vi "Read-Write Backspan Settings File.vi"(0 "configuration file path":path=path "C:/ProgramData/PVI Systems/Staple Inspection System/Measurement Settings.xml", 1 "Backplane Settings":T2={"Setup"={"Show Search Area"=FALSE, "Show Search Lines"=FALSE, "Show Edges Found"=FALSE, "Show Result"=FALSE}, "Outside Edge Options"={"Edge Polarity"=0, "Kernel Size"=13, "Width"=19, "Minimum Edge Strength"=100.0, "Interpolation Type"=enum."Zero Order", "Data Processing Method"=enum."Average"}, "Outside Line Options"={"Number of Lines"=1, "Type"=enum."First Edge Rake", "Min. Score"=0.0, "Max. Score"=1024.0, "Orientation"=0.0, "Angle Range"=40.0, "Angle Tolerance"=5.0, "Step Size"=20, "Min. SNR (db)"=0.0, "Min. Points (%)"=2.0, "Hough Iterations"=5}, "Settings Caliper"={"Contrast"=40, "Filter width"=4, "Steepness"=2, "Subsampling Ratio"=5, "Show Search Area"=FALSE, "Show Search Lines"=FALSE, "Show Edges Found"=FALSE, "Show Result"=FALSE}, "Look For (Bright Objects)"=1, "Method"=1, "Kernel Size"={"SizeX"=176, "SizeY"=176}, "Niblack Deviation Factor"=0.12, "Number of Erosion"=2, "Score Delineator"=150.0, "Auto Adjust Kernel Size"=TRUE, "Threshold Method"=0, "Use Quick method\nThreshold"=TRUE, "Scale Score"=TRUE, "Area Filter > 2"=10000.0, "Inside Edge Options"={"Edge Polarity"=1, "Kernel Size"=13, "Width"=19, "Minimum Edge Strength"=100.0, "Interpolation Type"=enum."Zero Order", "Data Processing Method"=enum."Average"}, "Inside Line Options"={"Number of Lines"=1, "Type"=enum."First Edge Rake", "Min. Score"=0.0, "Max. Score"=1024.0, "Orientation"=0.0, "Angle Range"=25.0, "Angle Tolerance"=1.0, "Step Size"=20, "Min. SNR (db)"=0.0, "Min. Points (%)"=1.0, "Hough Iterations"=5}, "Inner Width Reduce %"=5.0, "Inner Height Reduce %"=15.0, "Inner Setup"={"Show Search Area"=FALSE, "Show Search Lines"=FALSE, "Show Edges Found"=FALSE, "Show Result"=FALSE}, "Show CoM"=FALSE, "Keep All Results"=FALSE, "X Size"=0.0, "Y Size"=0.0, ">2 Holes % perimeter"=0.0, "Expected Backspan Width (Pixels)"=160, "Boundry Flex"=0.0, "Center Angle"=2.0} {"Inside Edge Options"."Edge Polarity" items=["All Edges", "Rising Edges", "Falling Edges"]; "Threshold Method" items=["clustering", "entropy", "metric", "moments", "inter-class variance"]; "Score Delineator" format="%#_15g"; "Niblack Deviation Factor" format="%#_15g"; "Method" items=["Niblack", "Background Correction"]; "Look For (Bright Objects)" items=["Bright Objects", "Dark Objects"]; "Outside Edge Options"."Edge Polarity" items=["All Edges", "Rising Edges", "Falling Edges"]}, 2 "Mode":T1=enum."Write", 3 "error in":errorcluster) -> (7 "Config File Path":path=path "C:/ProgramData/PVI Systems/Staple Inspection System/Config.ini", 8 "Backplane Settings Out":T2={"Setup"={"Show Search Area"=FALSE, "Show Search Lines"=FALSE, "Show Edges Found"=FALSE, "Show Result"=TRUE}, "Outside Edge Options"={"Edge Polarity"=0, "Kernel Size"=13, "Width"=19, "Minimum Edge Strength"=100.0, "Interpolation Type"=enum."Zero Order", "Data Processing Method"=enum."Average"}, "Outside Line Options"={"Number of Lines"=1, "Type"=enum."First Edge Rake", "Min. Score"=0.0, "Max. Score"=1024.0, "Orientation"=0.0, "Angle Range"=20.0, "Angle Tolerance"=1.0, "Step Size"=20, "Min. SNR (db)"=0.0, "Min. Points (%)"=2.0, "Hough Iterations"=5}, "Settings Caliper"={"Contrast"=40, "Filter width"=4, "Steepness"=2, "Subsampling Ratio"=5, "Show Search Area"=FALSE, "Show Search Lines"=FALSE, "Show Edges Found"=FALSE, "Show Result"=FALSE}, "Look For (Bright Objects)"=1, "Method"=1, "Kernel Size"={"SizeX"=176, "SizeY"=176}, "Niblack Deviation Factor"=0.2, "Number of Erosion"=2, "Score Delineator"=150.0, "Auto Adjust Kernel Size"=TRUE, "Threshold Method"=2, "Use Quick method\nThreshold"=TRUE, "Scale Score"=TRUE, "Area Filter > 2"=10000.0, "Inside Edge Options"={"Edge Polarity"=2, "Kernel Size"=13, "Width"=19, "Minimum Edge Strength"=100.0, "Interpolation Type"=enum."Zero Order", "Data Processing Method"=enum."Average"}, "Inside Line Options"={"Number of Lines"=1, "Type"=enum."First Edge Rake", "Min. Score"=0.0, "Max. Score"=1024.0, "Orientation"=0.0, "Angle Range"=25.0, "Angle Tolerance"=1.0, "Step Size"=20, "Min. SNR (db)"=0.0, "Min. Points (%)"=1.0, "Hough Iterations"=5}, "Inner Width Reduce %"=30.0, "Inner Height Reduce %"=15.0, "Inner Setup"={"Show Search Area"=FALSE, "Show Search Lines"=FALSE, "Show Edges Found"=FALSE, "Show Result"=TRUE}, "Show CoM"=FALSE, "Keep All Results"=FALSE, "X Size"=0.0, "Y Size"=0.0, ">2 Holes % perimeter"=0.0, "Expected Backspan Width (Pixels)"=140, "Boundry Flex"=0.0, "Center Angle"=0.0} {"Inside Edge Options"."Edge Polarity" items=["All Edges", "Rising Edges", "Falling Edges"]; "Threshold Method" items=["clustering", "entropy", "metric", "moments", "inter-class variance"]; "Score Delineator" format="%#_15g"; "Niblack Deviation Factor" format="%#_15g"; "Method" items=["Niblack", "Background Correction"]; "Look For (Bright Objects)" items=["Bright Objects", "Dark Objects"]; "Outside Edge Options"."Edge Polarity" items=["All Edges", "Rising Edges", "Falling Edges"]}, 10 "error out":errorcluster)   [LabVIEW 2013, in "Config Module.lvlib"]
uses:
  Config Module.lvlib
  Measurement Library/Controls/ASMS Backplane Settings Cluster.ctl
  Controls/Config File Operation Enum.ctl
  XML Config/XML Config.lvlib
  Measurement Library/Measurement Library.lvlib
panel:
  out "XML":string
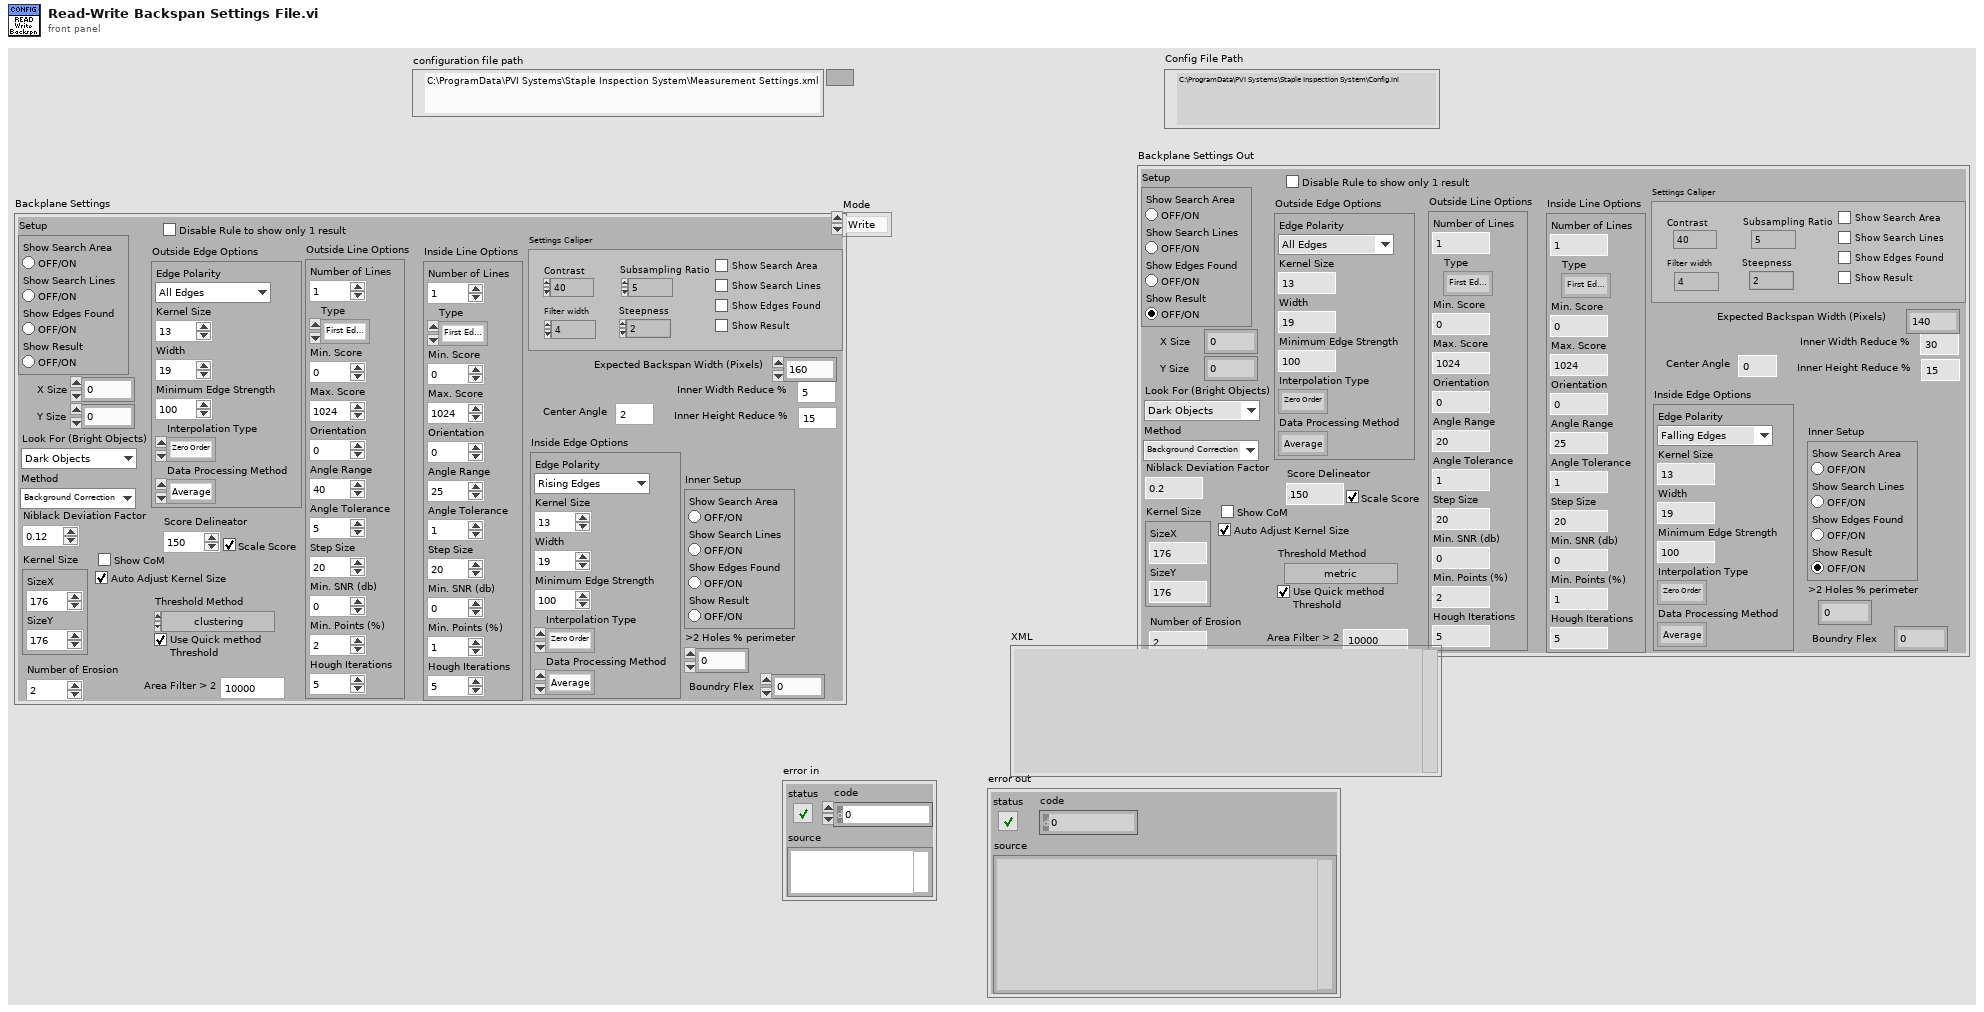
[diagram p1: front panel]
types:
  T1 = typedef "Config Module.lvlib/Config File Operation Enum.ctl" = enum16{"Read", "Write"}
  T2 = typedef "Measurement Library.lvlib/ASMS Backplane Settings Cluster.ctl" = cluster{"Setup":cluster{"Show Search Area":bool, "Show Search Lines":bool, "Show Edges Found":bool, "Show Result":bool}, "Outside Edge Options":cluster{"Edge Polarity":u32, "Kernel Size":u32, "Width":u32, "Minimum Edge Strength":sgl, "Interpolation Type":enum32{"Zero Order", "Bilinear", "Quadratic", "Cubic", "Bilinear Fixed"}, "Data Processing Method":enum32{"Average", "Median"}}, "Outside Line Options":cluster{"Number of Lines":i32, "Type":enum32{"First Edge Rake", "Best Edge Rake", "Hough Edge Rake", "First Edge Projection", "Best Edge Projection"}, "Min. Score":dbl, "Max. Score":dbl, "Orientation":dbl, "Angle Range":dbl, "Angle Tolerance":dbl, "Step Size":u32, "Min. SNR (db)":dbl, "Min. Points (%)":dbl, "Hough Iterations":i32}, "Settings Caliper":cluster{"Contrast":i32, "Filter width":i32, "Steepness":i32, "Subsampling Ratio":u32, "Show Search Area":bool, "Show Search Lines":bool, "Show Edges Found":bool, "Show Result":bool}, "Look For (Bright Objects)":u32, "Method":u32, "Kernel Size":cluster{"SizeX":i32, "SizeY":i32}, "Niblack Deviation Factor":dbl, "Number of Erosion":i32, "Score Delineator":dbl, "Auto Adjust Kernel Size":bool, "Threshold Method":i32, "Use Quick method\nThreshold":bool, "Scale Score":bool, "Area Filter > 2":dbl, "Inside Edge Options":cluster{"Edge Polarity":u32, "Kernel Size":u32, "Width":u32, "Minimum Edge Strength":sgl, "Interpolation Type":enum32{"Zero Order", "Bilinear", "Quadratic", "Cubic", "Bilinear Fixed"}, "Data Processing Method":enum32{"Average", "Median"}}, "Inside Line Options":cluster{"Number of Lines":i32, "Type":enum32{"First Edge Rake", "Best Edge Rake", "Hough Edge Rake", "First Edge Projection", "Best Edge Projection"}, "Min. Score":dbl, "Max. Score":dbl, "Orientation":dbl, "Angle Range":dbl, "Angle Tolerance":dbl, "Step Size":u32, "Min. SNR (db)":dbl, "Min. Points (%)":dbl, "Hough Iterations":i32}, "Inner Width Reduce %":dbl, "Inner Height Reduce %":dbl, "Inner Setup":cluster{"Show Search Area":bool, "Show Search Lines":bool, "Show Edges Found":bool, "Show Result":bool}, "Show CoM":bool, "Keep All Results":bool, "X Size":dbl, "Y Size":dbl, ">2 Holes % perimeter":dbl, "Expected Backspan Width (Pixels)":i32, "Boundry Flex":dbl, "Center Angle":dbl}
  T3 = enum16{"open", "replace", "create", "open or create", "replace or create", "replace or create with confirmation"}
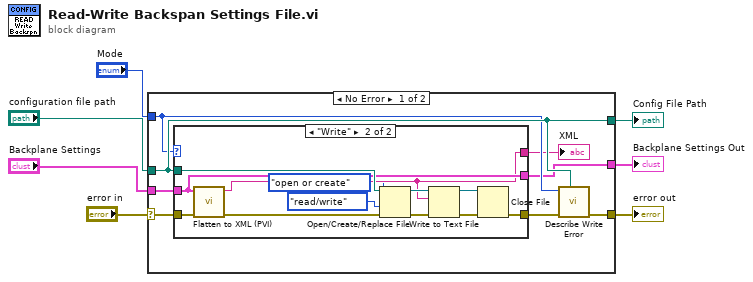
[diagram p0: block diagram]
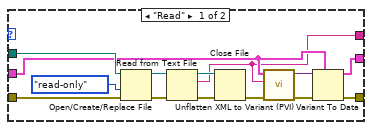
[diagram p2: hidden frame]
diagram:
  n1 = case shown="No Error" "error in" {
    selector: "error in" -> [w14 w43]
    tunnel: [w15 w43] -> w7
    tunnel: "configuration file path" -> [w13 w44]
    tunnel: "Backplane Settings" -> [w11 w42]
    tunnel: [w13 w44] -> w6
    tunnel: "Mode" -> [w12 _]
    tunnel: [w8 w42] -> w3
    frame No Error {
      n2 = case shown="\"Write\"" w12 {
        tunnel: w14 -> [w29 w36]
        tunnel: w13 -> [w24 w41]
        tunnel: w11 -> [w20 w37]
        tunnel: [w18 w34] -> w10
        tunnel: [w17 w31] -> w9
        tunnel: [w16 w37] -> w8
        frame "Read" {
          n3 = Open/Create/Replace File(file path (use dialog)=w24, error in=w29, access (0:read/write)=enum16{"read/write", "read-only", "write-only"}."read-only") -> (refnum out=w26:refnum<file>, error out=w28:errorcluster)  [unwired: 3 in, 1 out]
          n4 = Read from Text File(file (use dialog)=w26, error in=w28) -> (refnum out=w25:refnum<file>, text=w18:string, error out=w27:errorcluster)  [unwired: 2 in, 1 out]
          n5 = Close File(refnum=w25, error in=w27) -> (error out=w22:errorcluster)  [unwired: 1 out]
          n6 = call "Unflatten XML to Variant (PVI).vi"("error in (no error)"=w22, "XML"=w18, "Variant in (for type and default data)"=w20) -> ("error out"=w19:errorcluster, "Variant out"=w21:variant)  [unwired: 7 in]
          n7 = Variant To Data(error in=w19, type=w20, Variant=w21) -> (data=w16:T2, error out=w17:errorcluster)
        }
        frame "Write" {
          n8 = call "Flatten to XML (PVI).vi"("error in (no error)"=w36, "Variant"=w37) -> ("error out"=w35:errorcluster, "XML"=w34:string)  [unwired: 8 in]
          n9 = Open/Create/Replace File(file path (use dialog)=w41, error in=w35, operation (0:open)=T3."open or create", access (0:read/write)=enum16{"read/write", "read-only", "write-only"}."read/write") -> (refnum out=w39:refnum<file>, error out=w38:errorcluster)  [unwired: 2 in, 1 out]
          n10 = Write to Text File(file (use dialog)=w39, text=w34, error in=w38) -> (refnum out=w33:refnum<file>, error out=w32:errorcluster)  [unwired: 1 in, 1 out]
          n11 = Close File(refnum=w33, error in=w32) -> (error out=w31:errorcluster)  [unwired: 1 out]
        }
      }
      "XML" <- w10
      n12 = call "Describe Write Error.vi"("Config File Path"=w13, "error in (no error)"=w9, "Mode"=w12) -> ("error out"=w15:errorcluster)  [unwired: 8 in]
    }
    frame Error {
    }
  }
  "error out" <- w7
  "Config File Path" <- w6
  "Backplane Settings Out" <- w3
